vi "_ChangeMode.vi"(7 "refs":T3, 9 "Action in":T1 caption="Action", 10 "Display State In in":T5 caption="State", 11 "Data In in":T4) -> (0 "Position":T2, 1 "Action out":T1 caption="Action", 2 "Display State In out":T5 caption="State", 3 "Data In out":T4)   [LabVIEW 2013, in "UI_TimeSelector.xctl"]
uses:
  UI_TimeSelector.xctl
  State.ctl
  Typedefs/INTERNAL-DATA.ctl
  Interface/DEF-Mode.ctl
  Data.ctl
  Typedefs/INTERNAL-REFs.ctl
  <vilib>/Utility/miscctls.llb/LVRectTypeDef.ctl
  <vilib>/_xctls/Action.ctl
  <vilib>/_xctls/XControlSupport.lvlib
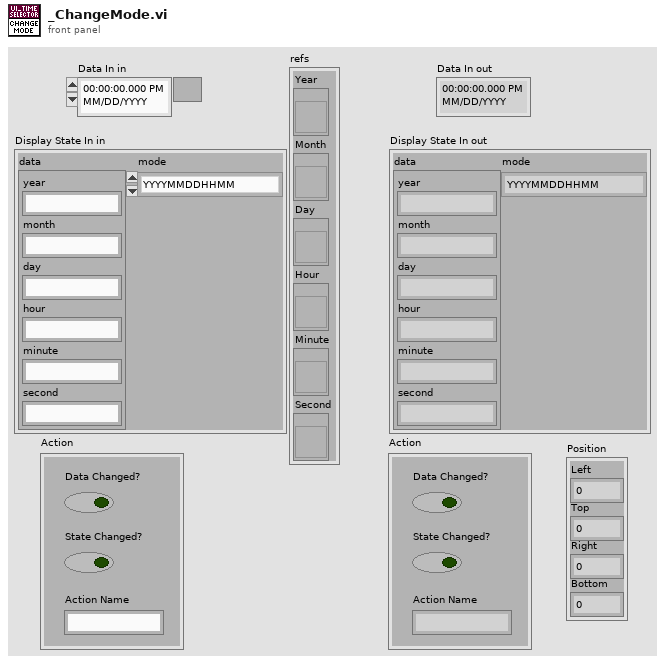
[diagram p1: front panel]
types:
  T1 = typedef "XControlSupport.lvlib/Action.ctl" = cluster{"Data Changed?":bool, "State Changed?":bool, "Action Name":string}
  T2 = typedef "LVRectTypeDef.ctl" = cluster{"Left":i16, "Top":i16, "Right":i16, "Bottom":i16}
  T3 = typedef "UI_TimeSelector.xctl/INTERNAL-REFs.ctl" = cluster{"Year":refnum<vi>, "Month":refnum<vi>, "Day":refnum<vi>, "Hour":refnum<vi>, "Minute":refnum<vi>, "Second":refnum<vi>}
  T4 = typedef "UI_TimeSelector.xctl/Data.ctl" = timestamp
  T5 = typedef "UI_TimeSelector.xctl/State.ctl" = cluster{"data":T6, "mode":T7}
  T6 = typedef "UI_TimeSelector.xctl/INTERNAL-DATA.ctl" = cluster{"year":string, "month":string, "day":string, "hour":string, "minute":string, "second":string}
  T7 = typedef "UI_TimeSelector.xctl/DEF-Mode.ctl" = enum16{"YYYYMMDDHHMM", "YYYYMMDDHHMMSS", "YYYY", "YYYYMM", "YYYYMMDD", "HHMM", "HHMMSS"}
  T8 = cluster{"Year":bool, "Month":bool, "Day":bool, "Hour":bool, "Minute":bool, "Second":bool}
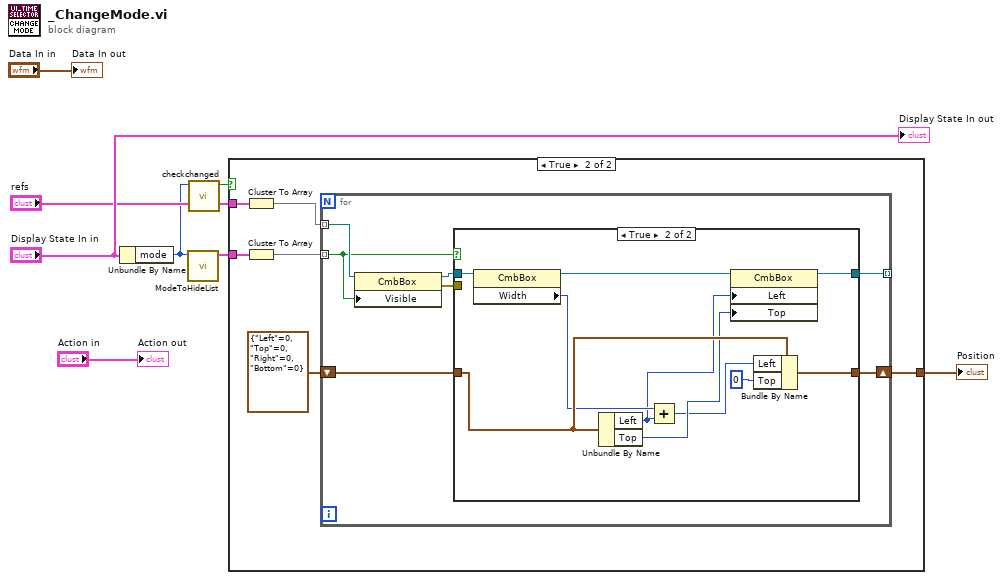
[diagram p0: block diagram]
diagram:
  n1 = Unbundle By Name("Display State In in") -> ("mode"=w3:T7)
  n2 = call "ModeToHideList.vi"("Value"=w3) -> ("mode"=w2:T8)  [unwired: 10 in]
  n3 = call "checkchanged.vi"("mode"=w3) -> ("Boolean"=w5:bool)  [unwired: 10 in]
  n4 = case shown="True" w5 {
    tunnel: "refs" -> [_ w14]
    tunnel: w2 -> [_ w11]
    tunnel: [_ w9] -> w4
    frame False {
    }
    frame True {
      n5 = Cluster To Array(cluster=w14) -> (array=w13:refnum<vi>[])
      n6 = Cluster To Array(cluster=w11) -> (array=w12:bool[])
      n7 = for {
        tunnel: w13 -> [w21] mode=indexing
        tunnel: w12 -> [w17] mode=indexing
        tunnel: [w18] -> _ mode=indexing
        shift-right: [w15] -> w9
        shift-left: T2 {"Left"=0, "Top"=0, "Right"=0, "Bottom"=0} ("Position") -> [w16]
        n8 = property class="CmbBox"(reference=w21, "Visible"=w17) -> (reference out=w20:refnum<vi>, error out=w19:errorcluster)  [unwired: 1 in]
        n9 = case shown="True" w17 {
          tunnel: w20 -> [w22 w30]
          tunnel: w19 -> [_ _]
          tunnel: [w22 w32] -> w18
          tunnel: w16 -> [w23 w31]
          tunnel: [w23 w33] -> w15
          frame False {
          }
          frame True {
            n10 = property class="CmbBox"(reference=w30) -> (reference out=w29:refnum<vi>, "Width"=w28:u32)  [unwired: 1 in, 1 out]
            n11 = Unbundle By Name(w31) -> ("Left"=w27:i16, "Top"=w26:i16)
            n12 = Add(x=w28, y=w27) -> (x+y=w25:u32)
            n13 = property class="CmbBox"(reference=w29, "Left"=w27, "Top"=w26) -> (reference out=w32:refnum<vi>)  [unwired: 1 in, 1 out]
            n14 = Bundle By Name(cluster=w31, "Left"=w25, "Top"=i16 0) -> (w33:T2)
          }
        }
      }
    }
  }
  "Position" <- w4
  "Display State In out" <- "Display State In in"
  "Data In out" <- "Data In in"
  "Action out" <- "Action in"
